vi "Write NumberOfRobots.vi"(8 "error in (no error)":errorcluster, 10 "NumberOfRobots":dbl=5.0, 11 "5RobotsKeeperGame in":refnum<class "5RobotsKeeperGame.lvclass">) -> (0 "error out":errorcluster, 3 "5RobotsKeeperGame out":refnum<class "5RobotsKeeperGame.lvclass">)   [LabVIEW 2020, in "5RobotsKeeperGame.lvclass"]
uses:
  5RobotsKeeperGame.lvclass
  5RobotsKeeperGame.lvclass/5RobotsKeeperGame.ctl
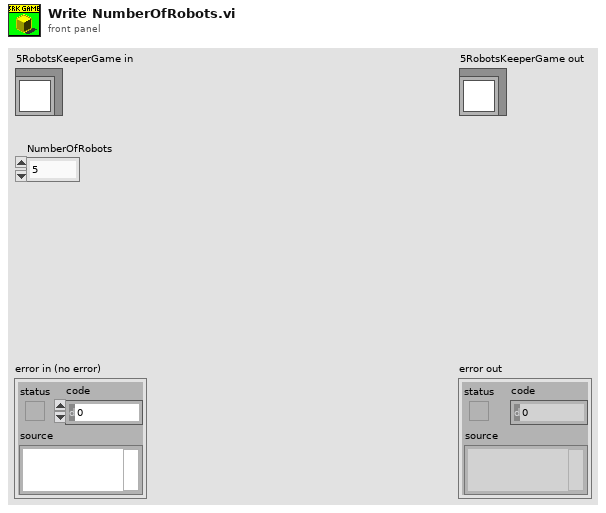
[diagram p1: front panel]
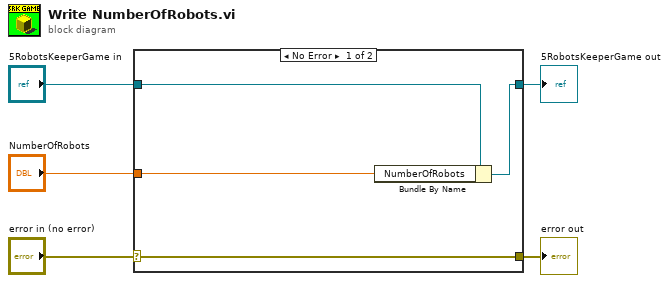
[diagram p0: block diagram]
diagram:
  n1 = case shown="No Error" "error in (no error)" {
    selector: "error in (no error)" -> [w9 w10]
    tunnel: [w9 w10] -> w4
    tunnel: [w7 w11] -> w2
    tunnel: "5RobotsKeeperGame in" -> [w8 w11]
    tunnel: "NumberOfRobots" -> [w6 _]
    frame No Error {
      n2 = Bundle By Name(cluster=w8, "NumberOfRobots"=w6) -> (w7:refnum<class "5RobotsKeeperGame.lvclass">)
    }
    frame Error {
    }
  }
  "error out" <- w4
  "5RobotsKeeperGame out" <- w2
